vi "Stop Core.vi"(10 "final error code":i32, 11 "CS++DIM-Server in":refnum<class "CS++DIM-Server.lvclass">) -> (3 "CS++DIM-Server out":refnum<class "CS++DIM-Server.lvclass">)   [LabVIEW 2015, in "CS++DIM-Server.lvlib" / "CS++DIM-Server.lvclass"]
doc: "(<B>Filename</B>: Actor Framework.lvlib:Actor.lvclass:Stop Core.vi)\n\nDefines what the actor does before it stops. Use the <B>final error code</B> input to determine whether the actor shut down in response to an error.\n\nBy default, this method does nothing. A descendant class may override it to define behavior, such as shutting down any processes the actor initiated in its override of the Actor Core method."
uses:
  CS++DIM-Server.lvclass
  CS++DIM-Server.lvclass/CS++DIM-Server.ctl
  CSPP_Core/Actors/CS++BaseActor/CS++BaseActor.lvclass
  CSPP_Core/Classes/CS++ProcessVariables/PVConnection/PVConnection.lvclass
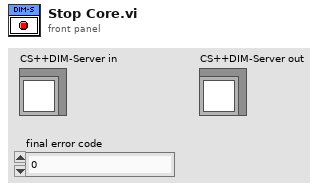
[diagram p1: front panel]
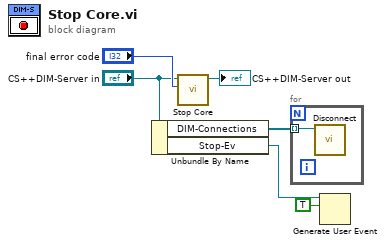
[diagram p0: block diagram]
diagram:
  n1 = Unbundle By Name("CS++DIM-Server in") -> ("DIM-Connections"=w3:refnum<class "PVConnection.lvclass">[], "Stop-Ev"=w2:refnum<user-event>)
  n2 = call-parent "Stop Core.vi"("final error code"="final error code", "CS++BaseActor in"="CS++DIM-Server in") -> ("CS++BaseActor out"=→"CS++DIM-Server out":refnum<class "CS++DIM-Server.lvclass">)  [unwired: 9 in]
  n3 = for {
    tunnel: w3 -> [w7] mode=indexing
    n4 = call "Disconnect.vi"("PVConnection in"=w7) -> ()  [unwired: 9 in, 2 out]
  }
  n5 = Generate User Event(user event=w2, event data cluster=TRUE ("event data")) -> ()  [unwired: 2 in, 2 out]
